vi "huntTic.vi"() -> ()   [LabVIEW 2021]
uses:
  <vilib>/Analysis/NI_AALBase.lvlib
  <vilib>/Analysis/1siggen.llb/Ramp Pattern by Delta.vi
  Tic/subVIs/TicProcedure.ctl
panel:
  in  "Stop":bool
  out "trying":u16
  in  "endAddress":u16=16384 max=16384
  out "Scaled Readback":dbl
  out "Error Out":errorcluster
  in  "Procedure":T1
  in  "Port Name (VISA)":refnum<visa-resource-name>
  in  "startAddress":u16=16384 max=16384
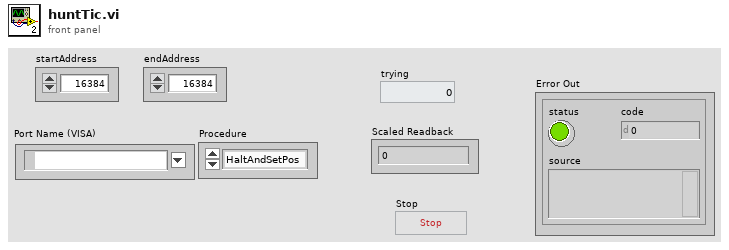
[diagram p1: front panel]
types:
  T1 = typedef "TicProcedure.ctl" = enum16{"HaltAndSetPos", "GetStatus", "GetPosition", "SetTarget", "GetTarget", "Enable", "Disable", "SetCurrent", "GetCurrent", "GetVelocity", "GetUptime", "GetVsupply", "Reset", "Go"}
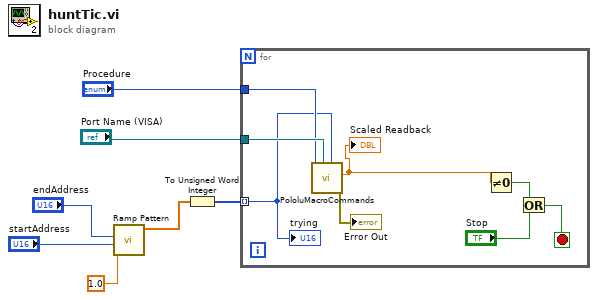
[diagram p0: block diagram]
diagram:
  n1 = call-poly <vilib>:"Ramp Pattern.vi"("start"="startAddress", "end"="endAddress", "delta"=1.0) -> ("Ramp Pattern"=w2:dbl[])  [unwired: 6 in, 2 out]
  n2 = To Unsigned Word Integer(number=w2) -> (unsigned 16bit integer=w1:u16[])
  n3 = for {
    tunnel: "Port Name (VISA)" -> [w15]
    tunnel: "Procedure" -> [w14]
    tunnel: w1 -> [w13] mode=indexing
    stop <- w8 stop-if-true
    n4 = call "PololuMacroCommands.vi"("Address"=w13, "Port Name (VISA)"=w15, "Procedure"=w14) -> ("Error Out"=→"Error Out":errorcluster, "Scaled Readback"=w11:dbl)  [unwired: 6 in, 1 out]
    "Scaled Readback" <- w11
    n5 = Not Equal To 0?(x=w11) -> (x != 0?=w10:bool)
    n6 = Or(x=w10, y="Stop") -> (x .or. y?=w8:bool)
    "trying" <- w13
  }
